vi "OpenCasperDrve4Motor.vi"(5 "ClimbRev":dbl, 7 "Encoder Ticks Per Rev":dbl, 9 "PID (Distance)":T1, 10 "PID (Speed)":T1) -> (0 "error out":errorcluster, 2 "Control Mode":T2)   [LabVIEW 2015]
uses:
  <vilib>/Rock Robotics/WPI/CAN/TalonSRX/WPI_CANTalonSRX_APIControlMode.ctl
  Advanced Drive VIs/PID Type Def.ctl
  LED Lights/Error Type Defs/Drive Error Type Def.ctl
  RobotDriveGlobal.vi
  LED Lights/LED Lights Global.vi
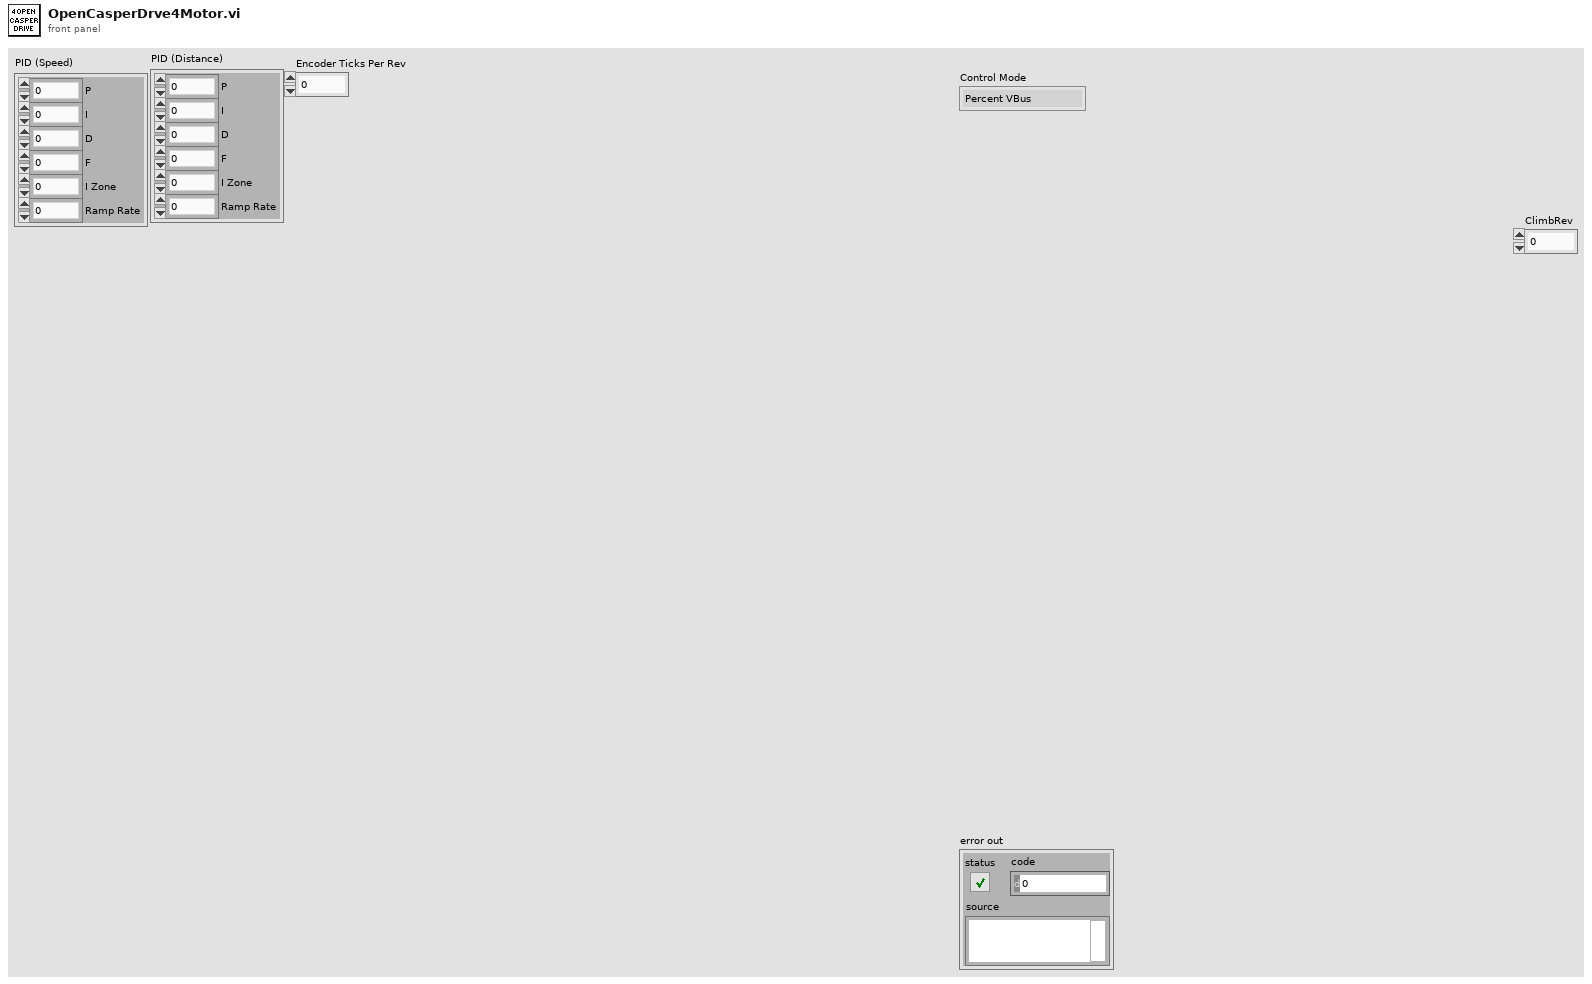
[diagram p1: front panel]
types:
  T1 = typedef "PID Type Def.ctl" = cluster{"P":dbl, "I":dbl, "D":dbl, "F":dbl, "I Zone":dbl, "Ramp Rate":dbl}
  T2 = typedef "WPI_CANTalonSRX_APIControlMode.ctl" = enum8{"Percent VBus", "Speed", "Position", "Slave", "Unchanged / Invalid", "Voltage Compensation", "Current", "Motion Profile"}
  T3 = typedef "Drive Error Type Def.ctl" = cluster{"Front Left":errorcluster, "Front Right":errorcluster, "Rear Left":errorcluster, "Rear Right":errorcluster}
  T4 = typedef "Drive Global Type Def.ctl" = cluster{"Left Drive Motors":T5, "Right Drive Motors":T5}
  T5 = typedef "Master Slave Drive Motors Type Def.ctl" = cluster{"Motor Front":T6, "Motor Back":T6, "Motor Errors":errorcluster, "Motor Top":T6, "Initialized":bool}
  T6 = typedef "Motor Global Type Def.ctl" = cluster{"Motor Error":errorcluster}
  T7 = typedef "WPI_MotorControlDeviceRef.ctl" = cluster{"DeviceStatus":errorcluster, "Type":T8, "PWM":cluster{"PWM Channel":T9, "DeadBand":T10}, "CAN":cluster{"Device Number":u8, "Control Mode":T11, "Semaphore":T12, "Max Vout":dbl, "TalonSRX Control Mode":T2}, "Invert":bool}
  T8 = typedef "WPI_MotorControlType.ctl" = enum16{"PWM", "CAN", "CANTalonSRX"}
  T9 = typedef "FPGA_DIOPWMChannel.ctl" = enum8{"PWM 0", "PWM 1", "PWM 2", "PWM 3", "PWM 4", "PWM 5", "PWM 6", "PWM 7", "PWM 8", "PWM 9", "PWM MXP 0", "PWM MXP 1", "PWM MXP 2", "PWM MXP 3", "PWM MXP 4", "PWM MXP 5", "PWM MXP 6", "PWM MXP 7", "PWM MXP 8", "PWM MXP 9", "Invalid"}
  T10 = typedef "WPI_PWMDeadband.ctl" = cluster{"Name":string, "maxPositivePwm":i32, "minPositivePwm":i32, "centerPwm":i32, "maxNegativePwm":i32, "minNegativePwm":i32, "angularRange":u16}
  T11 = typedef "WPI_CANJaguar_ControlMode.ctl" = enum8{"Percent VBus", "Current", "Speed", "Position", "Voltage"}
  T12 = typedef "Semaphore RefNum" = refnum<k1>
  T13 = typedef "RobotDrive Type Def.ctl" = cluster{"RobotDriveDevRef":cluster{"DevStatus":errorcluster, "Motors[]":T7[], "Square Inputs":bool, "Max Output":dbl}, "Control Mode":T2, "Motor Settings":T14, "Default Control Mode":T2, "Speed Mag":dbl}
  T14 = typedef "Drive Motor Settings.ctl" = cluster{"Wheel Radius":dbl, "Encoder Ticks Per Rev":dbl, "Gear Ratio":dbl, "ClimbRev":dbl}
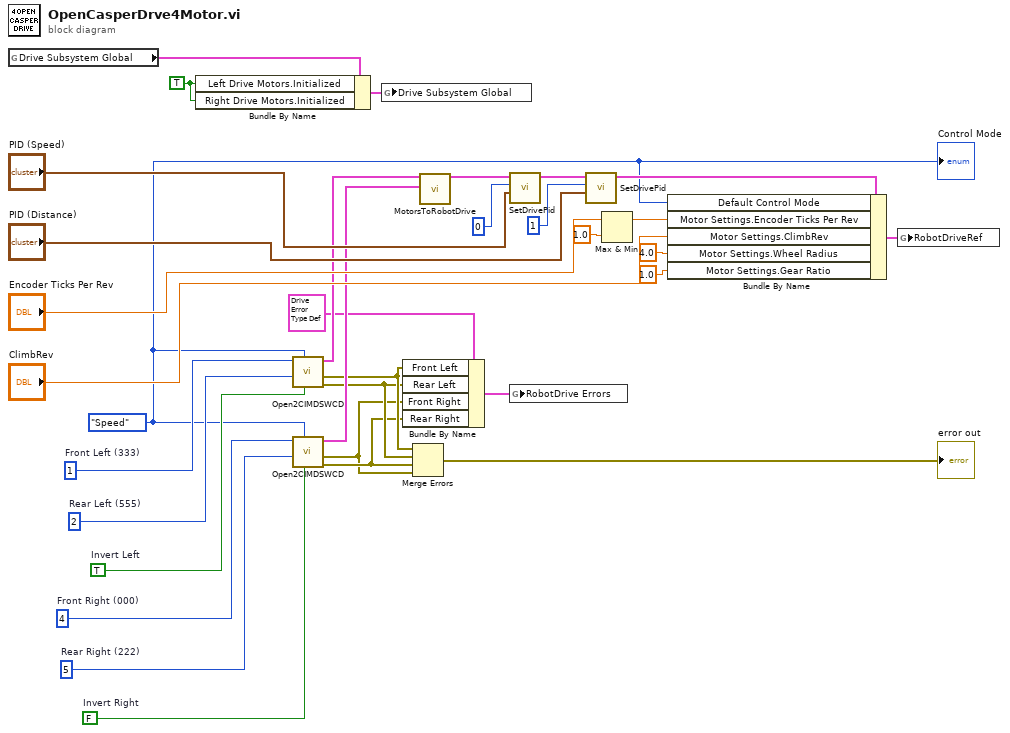
[diagram p0: block diagram]
diagram:
  w33 = TRUE
  w16 = FALSE  # Invert Right
  w17 = TRUE  # Invert Left
  w15 = u8 5  # Rear Right (222)
  w14 = u8 4  # Front Right (000)
  w18 = u8 2  # Rear Left (555)
  w19 = u8 1  # Front Left (333)
  w13 = WPI_CANTalonSRX_APIControlMode."Speed" ("Control Mode")
  n1 = global read "LED Lights Global.vi" "Drive Subsystem Global"() -> (w10:T4)
  n2 = Bundle By Name(cluster=w10, "Left Drive Motors.Initialized"=w33, "Right Drive Motors.Initialized"=w33) -> (w9:T4)
  n3 = call "Open2CIMDSWCD.vi"("Invert"=w17, "Control Mode"=w13, "Bottom Back"=w18, "Bottom Front"=w19) -> ("Back"=w3:errorcluster, "Front"=w4:errorcluster, "CAN Talon SRX Ref"=w12:T7)  [unwired: 5 in]
  n4 = call "Open2CIMDSWCD.vi"("Invert"=w16, "Control Mode"=w13, "Bottom Back"=w15, "Bottom Front"=w14) -> ("Back"=w2:errorcluster, "Front"=w1:errorcluster, "CAN Talon SRX Ref"=w11:T7)  [unwired: 5 in]
  n5 = global write "LED Lights Global.vi" "Drive Subsystem Global"(w9) -> ()
  n6 = Bundle By Name(cluster=T3 {"Front Left"={"status"=FALSE, "code"=0, "source"=""}, "Front Right"={"status"=FALSE, "code"=0, "source"=""}, "Rear Left"={"status"=FALSE, "code"=0, "source"=""}, "Rear Right"={"status"=FALSE, "code"=0, "source"=""}} ("RobotDrive Errors"), "Front Left"=w4, "Rear Left"=w3, "Front Right"=w1, "Rear Right"=w2) -> (w6:T3)
  n7 = Merge Errors(w4, w3, w2, w1) -> (→"error out":errorcluster)
  n8 = call "MotorsToRobotDrive.vi"("Left"=w12, "Right"=w11) -> ("RobotDriveRef"=w22:T13)  [unwired: 16 in, 1 out]
  n9 = call "SetDrivePid.vi"("PID"="PID (Speed)", "Profile Slot"=u8 0, "RobotDriveRef In"=w22) -> ("RobotDriveRef Out"=w30:T13)  [unwired: 7 in, 1 out]
  n10 = global write "RobotDriveGlobal.vi" "RobotDrive Errors"(w6) -> ()
  n11 = call "SetDrivePid.vi"("PID"="PID (Distance)", "Profile Slot"=u8 1, "RobotDriveRef In"=w30) -> ("RobotDriveRef Out"=w27:T13)  [unwired: 7 in, 1 out]
  n12 = Max & Min(x="Encoder Ticks Per Rev", y=1.0) -> (max(x,y)=w25:dbl)  [unwired: 1 out]
  n13 = Bundle By Name(cluster=w27, "Default Control Mode"=w13, "Motor Settings.Encoder Ticks Per Rev"=w25, "Motor Settings.ClimbRev"="ClimbRev", "Motor Settings.Wheel Radius"=4.0, "Motor Settings.Gear Ratio"=1.0) -> (w8:T13)
  n14 = global write "RobotDriveGlobal.vi" "RobotDriveRef"(w8) -> ()
  "Control Mode" <- w13
